vi "GetText.vi"(8 "error in":errorcluster, 11 "Getting Started IO editor node in":refnum<class "io editor node.lvclass">) -> (0 "error out":errorcluster, 1 "additional text":string, 2 "text":string, 3 "Getting Started IO editor node out":refnum<class "io editor node.lvclass">, 4 "glyph":string)   [LabVIEW 2015, in "io editor node.lvclass"]
uses:
  io editor node.lvclass
  <vilib>/NI/Tag Bus Data Framework/Configuration Editor/Classes/Module editor node/module editor node.lvclass
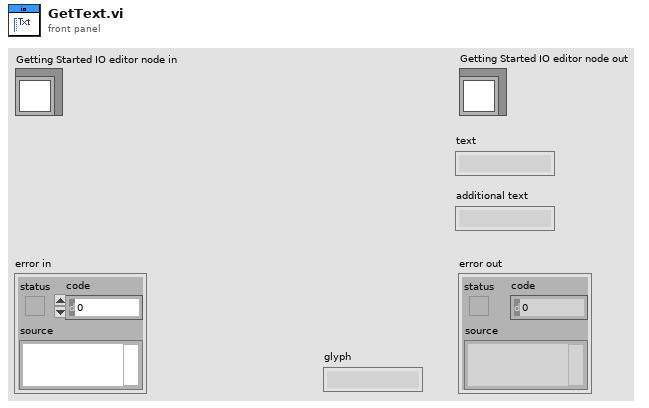
[diagram p1: front panel]
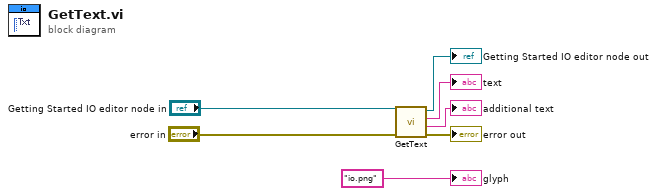
[diagram p0: block diagram]
diagram:
  n1 = call-parent "GetText.vi"("error in"="error in", "Module Editor Node in"="Getting Started IO editor node in") -> ("error out"=→"error out":errorcluster, "additional text"=→"additional text":string, "text"=→"text":string, "Module Editor Node out"=→"Getting Started IO editor node out":refnum<class "io editor node.lvclass">)  [unwired: 5 in, 1 out]
  "glyph" <- "io.png" ("glyph")
